vi "감지글로벌.vi"() -> ()   [LabVIEW 2020]
panel:
  out "감지 불리언":bool
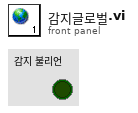
[diagram p1: front panel]
diagram:
